vi "Read Key Value - Double.vi"(4 "Default":dbl, 8 "error in (no error)":errorcluster, 9 "key":string, 10 "section":string, 11 "file refnum in":T1) -> (0 "error out":errorcluster, 2 "value":dbl, 3 "file refnum out":T1)   [LabVIEW 2019, in "TSC File IO.lvlib"]
doc: "This VI will read a section/key configuration file and return:\n<b>Double</b>\n\nInputs:\n-file refnum in [ref] - the reference to the open config file\n-section [string] - the section string in the configuration file\n-key [string] - the key to be read in the configuration file\n-error in\n\nOutputs:\n-file refnum out [ref] - the reference to the open config file\n-value [DBL] - the output data read\n-error out\n\n<b>Code Developed By:</b>\nDaniel Coons\nTechnology Service Corporation\n1983 S Liberty Drive\nBloomington, IN 47403\nwww.tsc.com\\atcs"
uses:
  TSC File IO.lvlib
  <vilib>/Utility/config.llb/Config Data RefNum.ctl
  <vilib>/Utility/config.llb/Read Key (Double).vi
  <vilib>/Utility/config.llb/NI_LVConfig.lvlib
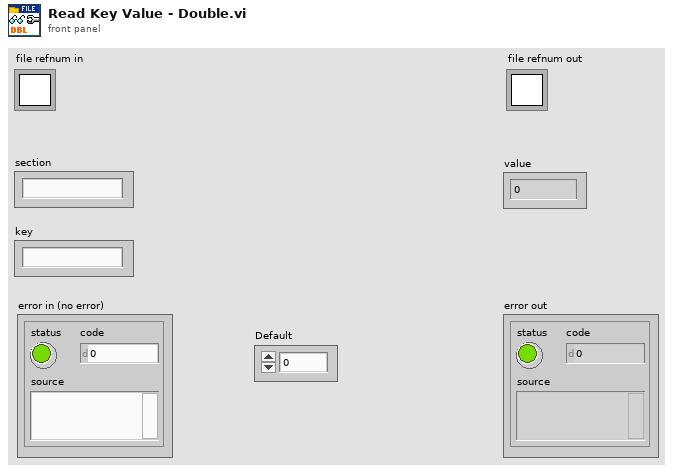
[diagram p1: front panel]
types:
  T1 = typedef "NI_LVConfig.lvlib/Config Data RefNum.ctl" = refnum<k1>
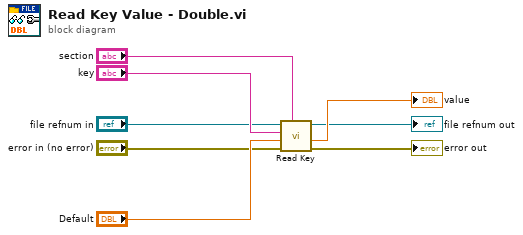
[diagram p0: block diagram]
diagram:
  n1 = call-poly <vilib>:"Read Key.vi"("section"="section", "error in (no error)"="error in (no error)", "default value"="Default", "key"="key", "refnum"="file refnum in") -> ("error out"=→"error out":errorcluster, "value"=→"value":dbl, "refnum out"=→"file refnum out":T1)  [unwired: 3 in, 1 out]
